vi "UART Receive.vi"(0 "UART Ref":T1={"FPGA I/O"="Mod1/DIO0", "Buffer Ref"="", "Stop Ref"=""}, 7 "Baud Rate (9600)":u32=9600) -> ()   [LabVIEW 2013, in "UART 8N1 (FPGA).lvlib"]
uses:
  UART 8N1 (FPGA).lvlib
  UART Ref.ctl
  RxD CMD.ctl
  <vilib>/Platform/TimedLoop/XDataNode/timing_clust.ctl
  <vilib>/Platform/TimedLoop/XDataNode/nitl_modes.ctl
  <vilib>/Platform/TimedLoop/XDataNode/wakeup.ctl
  <vilib>/rvi/Emulation/niFpgaSctlEmulationGetInTimedLoop.vi
  <vilib>/rvi/Emulation/niFpgaEmulationReportErrorSimple.vi
  <vilib>/rvi/Emulation/niFpgaGetClockAttributes.vi
  <vilib>/rvi/Emulation/niFpgaCriticalErrorInLSC.vi
  <vilib>/rvi/DataTransferAndStorage/Container/Common/niFpgaContainerExecOnDevCompGetState.vi
  <vilib>/rvi/DataTransferAndStorage/Register/Emulation/niFpgaRegisterEmulationFpgaImpl.vi
  <instcachedir>/0/niFpgaRegisterEmulationFpgaImpl_DCF4BC0110594B98B44A971D60CEEC4D.lvgen/niFpgaRegisterEmulationFpgaImpl_DCF4BC0110594B98B44A971D60CEEC4D_003.vi
  <vilib>/rvi/DataTransferAndStorage/Container/Common/niFpgaContainerGetUniqueNameForEmu.vi
  <vilib>/rvi/eio/common/nirviEmuTemplateMethod_errors.vi
  <vilib>/rvi/FIFO/Fifo_Resource/nirvififoEmulationWriteFpgaImpl.vi
  <vilib>/rvi/interface/RandomDataEmulation/nirviRandomDataFPGAFIFO.vi
  <vilib>/rvi/interface/RandomDataEmulation/niFpgaRandomDataHandleErrors.vi
  <vilib>/rvi/eio/common/nirviEmuReportErrorAndStop.vi
  <vilib>/rvi/FIFO/Fifo_Resource/nirvififoEmulationClearFpgaImpl.vi
  <vilib>/Platform/TimedLoop/XDataNode/XDataNode.xnode
  <vilib>/rvi/DataTransferAndStorage/Container/XNode/niFpgaContainer.xnode
  <vilib>/rvi/DataTransferAndStorage/Register/Emulation/niFpgaRegisterEmulationRefIn.vi
  <vilib>/eio/EIONode/EIONode.xnode
  <vilib>/rvi/FIFO/Fifo_Resource/niFpgaFifoEmulationRefIn.vi
  <vilib>/Platform/TimedLoop/XDataNode/XDNodeRunTimeDep.lvlib
panel:
  out "Receive Buffer Overflow":bool
  # "UART Receive\nRxD, 8N1"
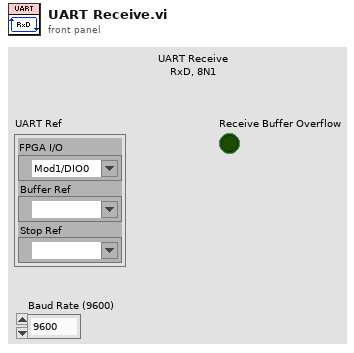
[diagram p1: front panel]
types:
  T1 = typedef "UART 8N1 (FPGA).lvlib/UART Ref.ctl" = cluster{"FPGA I/O":refnum<k21>, "Buffer Ref":refnum<k21>, "Stop Ref":refnum<k21>}
  T2 = typedef "UART 8N1 (FPGA).lvlib/RxD CMD.ctl" = enum16{"Init", "Wait on Falling Edge", "Wait Half Bit", "Wait One Bit", "Read Data Bit", "Wait Stop Time", "Close"}
  T3 = typedef "XDNodeRunTimeDep.lvlib/timing_clust.ctl" = cluster{"Expected End [f-1]":u64, "Actual End [f-1]":u64, "Finished Late? [f-1]":bool, "Expected End [i-1]":u64, "Actual End [i-1]":u64, "Finished Late? [i-1]":bool, "Expected Start [i]":u64, "Actual Start [i]":u64, "Expected Start [f]":u64, "Actual Start [f]":u64, "Source Name":string, "Structure Name":string, "Period":i64, "Deadline":i64, "Offset":i64, "Start":i64, "Priority":i32, "Timeout":i32, "Mode":T4, "Wakeup Reason":T5, "Error":errorcluster, "Source Type":string, "Secondary Source Type":string, "Global End Time":u64, "Global Start Time":u64, "Frame Duration":u64, "Iteration Duration":u64, "Assigned CPU":i32, "I/O Scan Engine Mode":u32}
  T4 = typedef "XDNodeRunTimeDep.lvlib/nitl_modes.ctl" = enum32{"No Change", "Process missed periods, maintain original phase", "Discard missed periods, maintain original phase", "Process missed periods, ignore original phase", "Discard missed periods, ignore original phase"}
  T5 = typedef "XDNodeRunTimeDep.lvlib/wakeup.ctl" = enum32{"Normal", "Aborted", "Asynchronous wakeup", "Timing source error", "Timed loop error", "Timeout"}
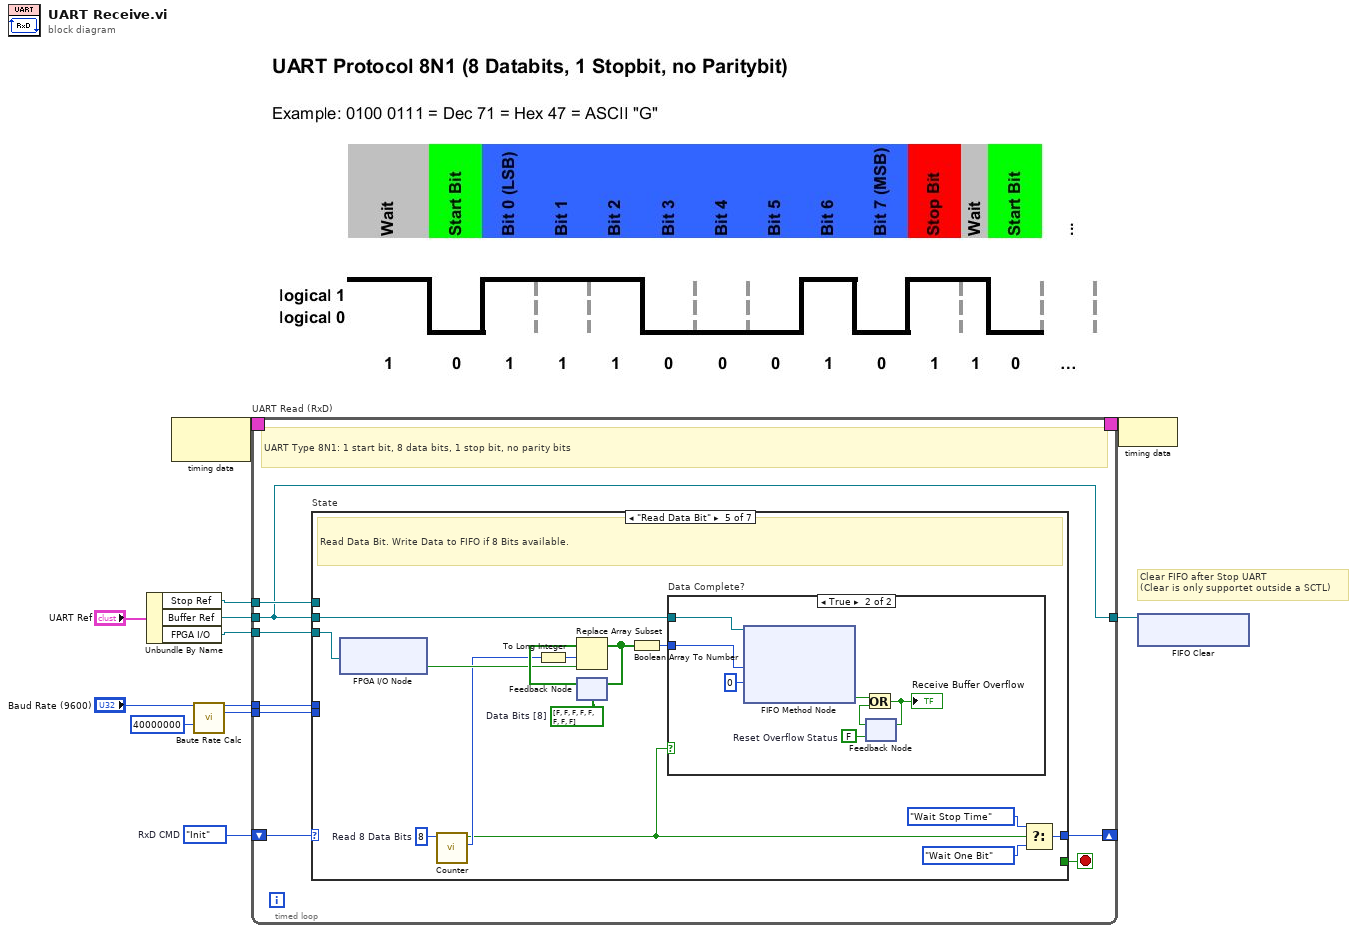
[diagram p0: block diagram]
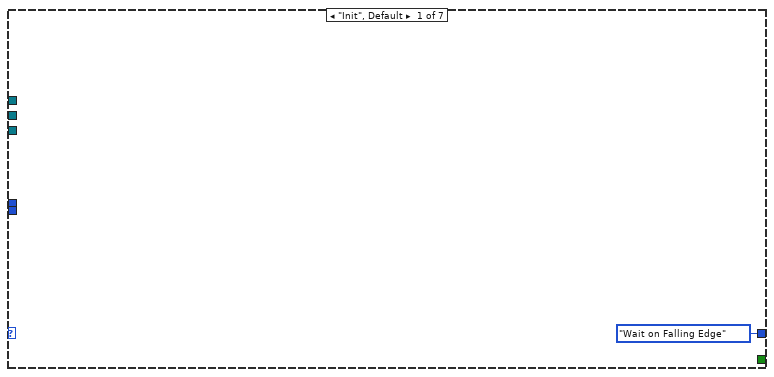
[diagram p2: hidden frame]
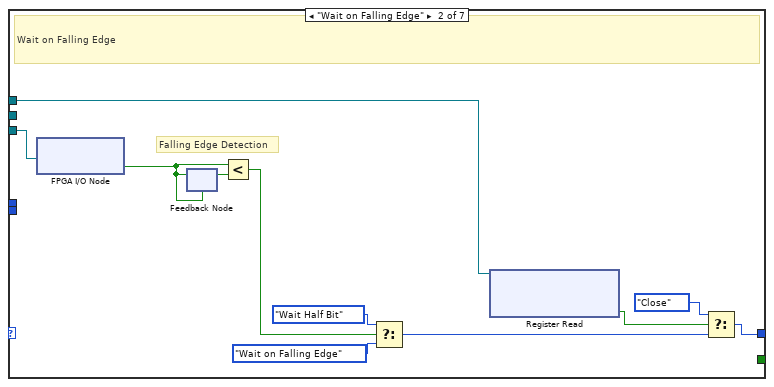
[diagram p3: hidden frame]
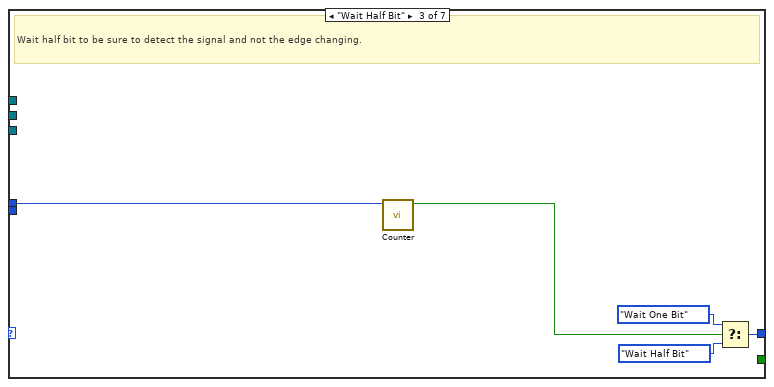
[diagram p4: hidden frame]
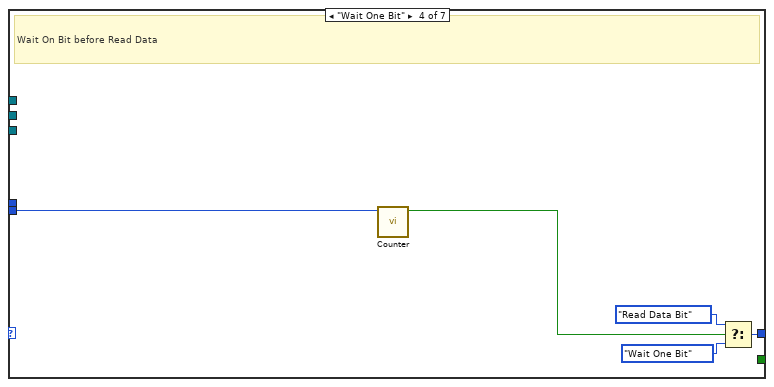
[diagram p5: hidden frame]
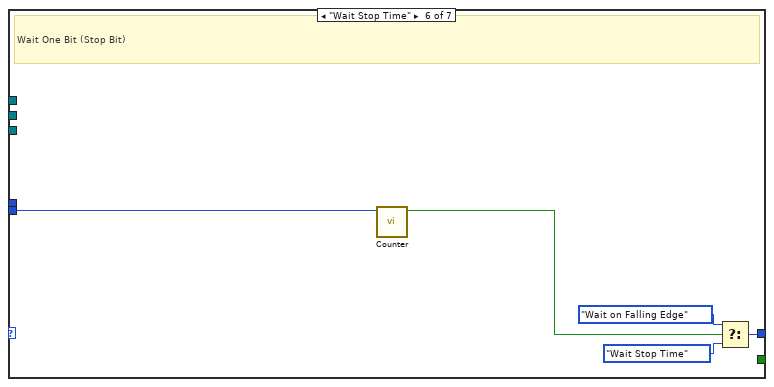
[diagram p7: hidden frame]
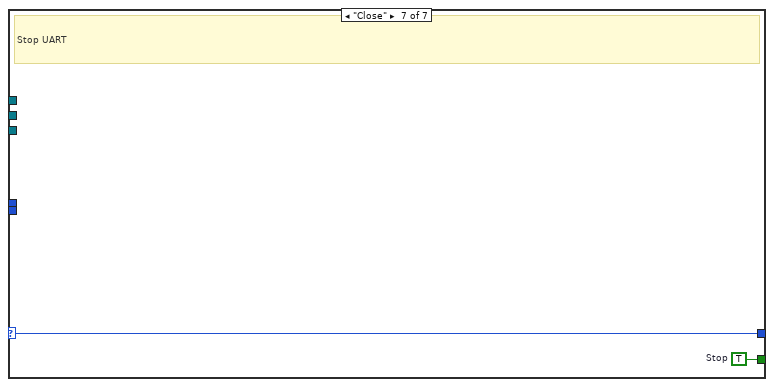
[diagram p8: hidden frame]
diagram:
  w10 = RxD_CMD."Init"  # RxD CMD
  # "Clear FIFO after Stop UART\n(Clear is only supportet outside a SCTL)"
  n1 = Unbundle By Name("UART Ref") -> ("Stop Ref"=w6:refnum<k21>, "Buffer Ref"=w8:refnum<k21>, "FPGA I/O"=w9:refnum<k21>)
  n2 = node-c288() -> (w12:T3)  [unwired: 1 in]
  n3 = call "Baute Rate Calc.vi"("Baud Rate (9600)"="Baud Rate (9600)", "FPGA Clock Rate (40000000)"=u32 40000000) -> ("Half Bit"=w4:u32, "One Bit"=w3:u32)  [unwired: 10 in, 2 out]
  n4 = timed-loop "UART Read (RxD)" {
    timing: w12 -> [_]
    timing-out: [_] -> w11
    shift-right: [w18] -> _
    shift-left: w10 -> [w15]
    tunnel: w4 -> [w17]
    tunnel: w9 -> [w20]
    tunnel: w3 -> [w16]
    tunnel: w8 -> [w13]
    tunnel: w6 -> [w14]
    tunnel: [w13] -> w5
    stop <- w19 stop-if-true
    # "UART Type 8N1: 1 start bit, 8 data bits, 1 stop bit, no parity bits"
    n5 = case "State" shown="\"Wait on Falling Edge\"" w15 {
      selector: w15 -> [_ _ _ _ _ _ w69]
      tunnel: w20 -> [_ w32 _ _ w56 _ _]
      tunnel: [_ _ _ _ _ _ w70] -> w19
      tunnel: [RxD_CMD."Wait on Falling Edge" ("RxD State") w24 w35 w39 w48 w65 w69] -> w18
      tunnel: w17 -> [_ _ w33 _ _ _ _]
      tunnel: w16 -> [_ _ _ w38 _ w64 _]
      tunnel: w13 -> [_ _ _ _ w43 _ _]
      tunnel: w14 -> [_ w23 _ _ _ _ _]
      frame "Init", Default {
      }
      frame "Wait on Falling Edge" {
        # "Falling Edge Detection"
        # "Wait on Falling Edge"
        n6 = xnode "FPGA I/O Node"("FPGA I/O In"=w32) -> ("I/O Item"=w30:bool)  [unwired: 1 out]
        n7 = feedback #1(w30) -> (w31:bool)
        n8 = feedback-in #1(w30) -> ()
        n9 = Less?(x=w30, y=w31) -> (x < y?=w29:bool)
        n10 = Select(t=RxD_CMD."Wait Half Bit", s=w29, f=RxD_CMD."Wait on Falling Edge" ("RxD State")) -> (s? t:f=w25:T2)
        n11 = xnode ("Register Read")("Register In"=w23) -> ("Data"=w22:bool)  [unwired: 1 out]
        n12 = Select(t=RxD_CMD."Close", s=w22, f=w25) -> (s? t:f=w24:T2)
      }
      frame "Wait Half Bit" {
        # "Wait half bit to be sure to detect the signal and not the edge changing."
        n13 = call "Counter.vi"("Counter End  Value"=w33) -> ("End Reached"=w34:bool)  [unwired: 9 in, 1 out]
        n14 = Select(t=RxD_CMD."Wait One Bit", s=w34, f=RxD_CMD."Wait Half Bit" ("RxD State")) -> (s? t:f=w35:T2)
      }
      frame "Wait One Bit" {
        # "Wait On Bit before Read Data"
        n15 = call "Counter.vi"("Counter End  Value"=w38) -> ("End Reached"=w42:bool)  [unwired: 9 in, 1 out]
        n16 = Select(t=RxD_CMD."Read Data Bit", s=w42, f=RxD_CMD."Wait One Bit" ("RxD State")) -> (s? t:f=w39:T2)
      }
      frame "Read Data Bit" {
        w44 = u32 8  # Read 8 Data Bits
        w55 = bool[] [FALSE, FALSE, FALSE, FALSE, FALSE, FALSE, FALSE, FALSE]  # Data Bits [8]
        # "Read Data Bit. Write Data to FIFO if 8 Bits available."
        n17 = xnode "FPGA I/O Node"("FPGA I/O In"=w56) -> ("I/O Item"=w53:bool)  [unwired: 1 out]
        n18 = call "Counter.vi"("Counter End  Value"=w44) -> ("Counter Value"=w52:u32, "End Reached"=w46:bool)  [unwired: 9 in]
        n19 = To Long Integer(number=w52) -> (32bit integer=w51:i32)
        n20 = feedback #2(w55) -> (w54:bool[])
        n21 = Replace Array Subset(array=w54, new element=w53, index=w51) -> (w47:bool[])
        n22 = feedback-in #2(w47) -> ()
        n23 = Boolean Array To Number(Boolean array=w47) -> (number=w45:u8)
        n24 = case "Data Complete?" shown="True" w46 {
          tunnel: w45 -> [_ w63]
          tunnel: w43 -> [_ w57]
          frame False {
          }
          frame True {
            w59 = FALSE  # Reset Overflow Status
            n25 = xnode ("FIFO Method Node")("Element"=w63, "Timeout"=0, "FIFO In"=w57) -> ("Timed Out?"=w62:bool)  [unwired: 1 out]
            n26 = feedback #3(w59) -> (w60:bool)
            n27 = Or(x=w62, y=w60) -> (x .or. y?=w61:bool)
            "Receive Buffer Overflow" <- w61
            n28 = feedback-in #3(w61) -> ()
          }
        }
        n29 = Select(t=RxD_CMD."Wait Stop Time", s=w46, f=RxD_CMD."Wait One Bit" ("RxD State")) -> (s? t:f=w48:T2)
      }
      frame "Wait Stop Time" {
        # "Wait One Bit (Stop Bit)"
        n30 = call "Counter.vi"("Counter End  Value"=w64) -> ("End Reached"=w66:bool)  [unwired: 9 in, 1 out]
        n31 = Select(t=RxD_CMD."Wait on Falling Edge", s=w66, f=RxD_CMD."Wait Stop Time" ("RxD State")) -> (s? t:f=w65:T2)
      }
      frame "Close" {
        w70 = TRUE  # Stop
        # "Stop UART"
      }
    }
  }
  n32 = node-c288(w11) -> ()
  n33 = xnode ("FIFO Clear")("FIFO In"=w5) -> ()  [unwired: 1 out]
